vi "NN_Torque_Allocator.vi"(1 "Inputs":dbl[](array[numeric])) -> (0 "Output":dbl[](array[numeric]))   [LabVIEW 2023]
uses:
  <vilib>/Analysis/baseanly.llb/A x Vector.vi
  NN_model_params.vi
  <vilib>/Analysis/NI_AALBase.lvlib
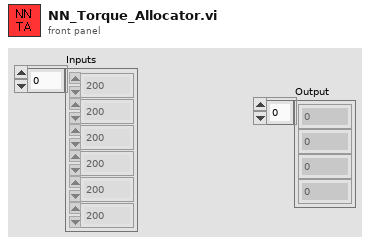
[diagram p1: front panel]
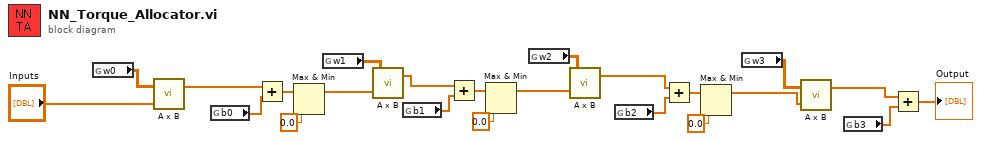
[diagram p0: block diagram]
diagram:
  n1 = global read "NN_model_params.vi" "w0"() -> (w12:sgl[][])
  n2 = call-poly <vilib>:"A x B.vi"("Vector"="Inputs", "A"=w12) -> ("A x Vector"=w23:dbl[])  [unwired: 1 out]
  n3 = global read "NN_model_params.vi" "b0"() -> (w9:sgl[])
  n4 = Add ("Add.vi")(x=w23, y=w9) -> (x+y=w21:dbl[])
  n5 = Max & Min(x=w21, y=0.0) -> (max(x,y)=w15:dbl[])  [unwired: 1 out]
  n6 = global read "NN_model_params.vi" "w1"() -> (w11:sgl[][])
  n7 = call-poly <vilib>:"A x B.vi"("Vector"=w15, "A"=w11) -> ("A x Vector"=w14:dbl[])  [unwired: 1 out]
  n8 = global read "NN_model_params.vi" "b1"() -> (w8:sgl[])
  n9 = Add ("Add.vi")(x=w14, y=w8) -> (x+y=w19:dbl[])
  n10 = Max & Min(x=w19, y=0.0) -> (max(x,y)=w13:dbl[])  [unwired: 1 out]
  n11 = global read "NN_model_params.vi" "w2"() -> (w10:sgl[][])
  n12 = call-poly <vilib>:"A x B.vi"("Vector"=w13, "A"=w10) -> ("A x Vector"=w6:dbl[])  [unwired: 1 out]
  n13 = global read "NN_model_params.vi" "b2"() -> (w7:sgl[])
  n14 = Add ("Add.vi")(x=w6, y=w7) -> (x+y=w17:dbl[])
  n15 = Max & Min(x=w17, y=0.0) -> (max(x,y)=w4:dbl[])  [unwired: 1 out]
  n16 = global read "NN_model_params.vi" "w3"() -> (w5:sgl[][])
  n17 = call-poly <vilib>:"A x B.vi"("Vector"=w4, "A"=w5) -> ("A x Vector"=w3:dbl[])  [unwired: 1 out]
  n18 = global read "NN_model_params.vi" "b3"() -> (w2:sgl[])
  n19 = Add(x=w3, y=w2) -> (x+y=→"Output":dbl[])
